vi "Magnitude.vi"(8 "error in (no error)":errorcluster, 11 "SnailNum in":refnum<class "SnailNum.lvclass">) -> (0 "error out":errorcluster, 2 "Magnitude":i64, 3 "SnailNum out":refnum<class "SnailNum.lvclass">)   [LabVIEW 2020, in "SnailNum.lvclass"]
uses:
  SnailNum.lvclass
  SnailNum.lvclass/SnailNum.ctl
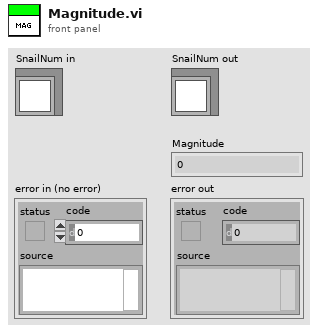
[diagram p1: front panel]
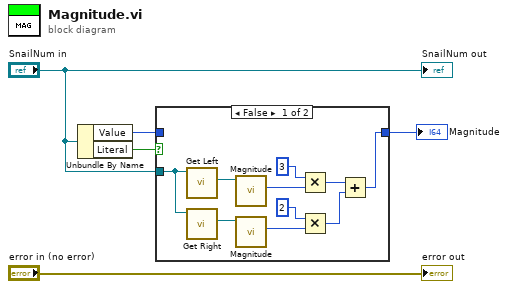
[diagram p0: block diagram]
diagram:
  n1 = Unbundle By Name("SnailNum in") -> ("Value"=w3:i64, "Literal"=w4:bool)
  n2 = case shown="False" w4 {
    tunnel: w3 -> [_ w16]
    tunnel: [w6 w16] -> w2
    tunnel: "SnailNum in" -> [w15 _]
    frame False {
      n3 = call "Get Left.vi"("SnailNum in"=w15) -> ("Left"=w13:refnum<class "SnailNum.lvclass">)  [unwired: 8 in, 2 out]
      n4 = call "Get Right.vi"("SnailNum in"=w15) -> ("Right"=w14:refnum<class "SnailNum.lvclass">)  [unwired: 8 in, 2 out]
      n5 = call "Magnitude.vi"("SnailNum in"=w13) -> ("Magnitude"=w12:i64)  [unwired: 8 in, 2 out]
      n6 = call "Magnitude.vi"("SnailNum in"=w14) -> ("Magnitude"=w10:i64)  [unwired: 8 in, 2 out]
      n7 = Multiply(x=i64 3, y=w12) -> (x*y=w8:i64)
      n8 = Multiply(x=i64 2, y=w10) -> (x*y=w7:i64)
      n9 = Add(x=w8, y=w7) -> (x+y=w6:i64)
    }
    frame True {
    }
  }
  "Magnitude" <- w2
  "error out" <- "error in (no error)"
  "SnailNum out" <- "SnailNum in"
